vi "Display Array.vi"(0 "output array":dbl[](array[numeric])) -> (4 "output array 2":dbl[](array[numeric]))   [LabVIEW 2013]
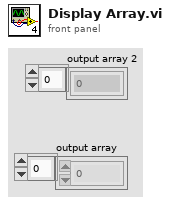
[diagram p1: front panel]
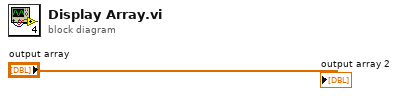
[diagram p0: block diagram]
diagram:
  "output array 2" <- "output array"
